vi "Harv_2_9.vi"(6 "Harvest":bool, 7 "Fire":bool, 8 "FireBallSen":bool, 9 "BallAcquired":bool, 10 "HarvPot":dbl, 11 "HarvSetpoints":dbl[](array[numeric])) -> (0 "HarvCleared":bool, 2 "HarvRoller":dbl, 3 "HarvPower":dbl)   [LabVIEW 2013]
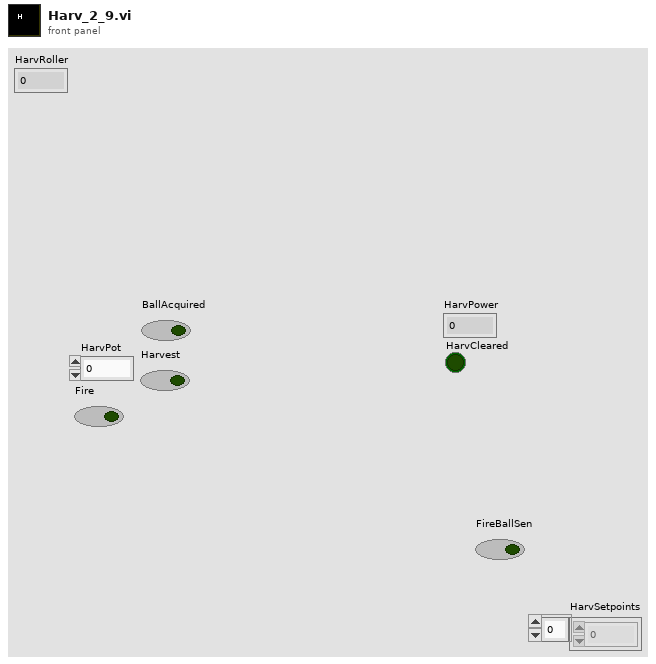
[diagram p1: front panel]
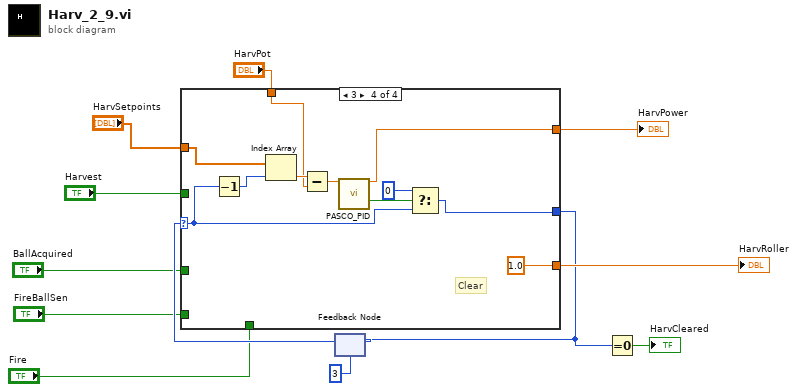
[diagram p0: block diagram]
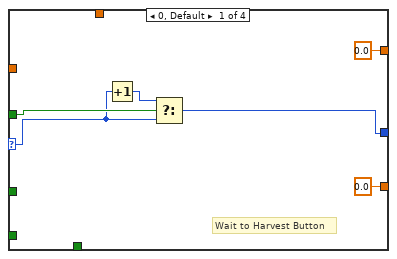
[diagram p2: hidden frame]
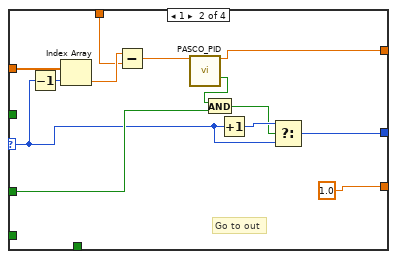
[diagram p3: hidden frame]
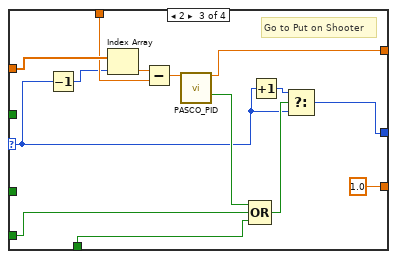
[diagram p4: hidden frame]
diagram:
  n1 = feedback #1(3 ("Numeric")) -> (w9:i32)
  n2 = case shown="3" w9 {
    selector: w9 -> [w13 w19 w32 w46]
    tunnel: "HarvSetpoints" -> [_ w31 w44 w55]
    tunnel: "HarvPot" -> [_ w29 w42 w54]
    tunnel: [0.0 ("Output") w27 w40 w52] -> w10
    tunnel: [w15 w25 w39 w50] -> w3
    tunnel: [0.0 1.0 1.0 1.0] -> w8
    tunnel: "BallAcquired" -> [_ w21 _ _]
    tunnel: "FireBallSen" -> [_ _ w35 _]
    tunnel: "Fire" -> [_ _ w34 _]
    tunnel: "Harvest" -> [w16 _ _ _]
    frame 0, Default {
      # "Wait to Harvest Button"
      n3 = Increment(x=w13) -> (x+1=w14:i32)
      n4 = Select(t=w14, s=w16, f=w13) -> (s? t:f=w15:i32)
    }
    frame 1 {
      # "Go to out"
      n5 = Decrement(x=w19) -> (x-1=w20:i32)
      n6 = Index Array(array=w31, index=w20) -> (element=w30:dbl)
      n7 = Subtract(x=w30, y=w29) -> (x-y=w28:dbl)
      n8 = call "PASCO_PID.vi"("Delta"=w28) -> ("Output"=w27:dbl, "IsThere"=w23:bool)  [unwired: 13 in]
      n9 = And(x=w23, y=w21) -> (x .and. y?=w22:bool)
      n10 = Increment(x=w19) -> (x+1=w26:i32)
      n11 = Select(t=w26, s=w22, f=w19) -> (s? t:f=w25:i32)
    }
    frame 2 {
      # "Go to Put on Shooter"
      n12 = Decrement(x=w32) -> (x-1=w33:i32)
      n13 = Index Array(array=w44, index=w33) -> (element=w43:dbl)
      n14 = Subtract(x=w43, y=w42) -> (x-y=w41:dbl)
      n15 = call "PASCO_PID.vi"("Delta"=w41) -> ("Output"=w40:dbl, "IsThere"=w36:bool)  [unwired: 13 in]
      n16 = Compound Arithmetic op=OR(w36, w35, w34) -> (w37:bool)
      n17 = Increment(x=w32) -> (x+1=w38:i32)
      n18 = Select(t=w38, s=w37, f=w32) -> (s? t:f=w39:i32)
    }
    frame 3 {
      # "Clear"
      n19 = Decrement(x=w46) -> (x-1=w47:i32)
      n20 = Index Array(array=w55, index=w47) -> (element=w56:dbl)
      n21 = Subtract(x=w56, y=w54) -> (x-y=w53:dbl)
      n22 = call "PASCO_PID.vi"("Delta"=w53) -> ("Output"=w52:dbl, "IsThere"=w51:bool)  [unwired: 13 in]
      n23 = Select(t=0, s=w51, f=w46) -> (s? t:f=w50:i32)
    }
  }
  "HarvRoller" <- w8
  "HarvPower" <- w10
  n24 = feedback-in #1(w3) -> ()
  n25 = Equal To 0?(x=w3) -> (x = 0?=→"HarvCleared":bool)
